vi "Numeric Functions.vi"() -> ()   [LabVIEW 2023]
doc: "This example shows how the Add function operates with different data types. These concepts also apply to the Subtract, Multiply, and Divide, Increment, Decrement, Add Array Elements, Multiply Array Elements, Absolute Value, Round To Nearest, Round To -Infinity, Round To +Infinity, Scale By Power, Square Root, Square, Negate, Reciprocal, and Sign functions."
uses:
  <vilib>/silver_ctls/ArrayMatrixCluster/Real Matrix NI_Silver.ctl
  <vilib>/Analysis/Matrix/Numeric/Add/Add - RM,RM.vi
  <vilib>/Analysis/Matrix/NI_Matrix.lvlib
panel:
  in  "Tab Control":T1(tab)
  in  "Numeric Addend 2":dbl=2.0
  in  "Numeric Addend 1":dbl=1.0
  out "Numeric Sum":dbl
  out "Array Sum":dbl[](array[numeric])
  in  "Array Addend 2":dbl[](array[numeric])=[10.0, 11.0, 12.0, 13.0]
  in  "Array Addend 1":dbl[](array[numeric])=[0.0, 1.0, 2.0]
  out "Array Sum":dbl[](array[numeric])
  in  "Array Addend":dbl[](array[numeric])=[0.0, 1.0, 2.0]
  in  "Numeric Addend":dbl=10.0
  out "Real Matrix Sum":T2
  in  "Real Matrix Addend 2":T2=[[10.0, 11.0, 12.0], [13.0, 14.0, 15.0], [16.0, 17.0, 18.0]]
  in  "Real Matrix Addend 1":T2=[[0.0, 1.0, 2.0], [3.0, 4.0, 5.0], [6.0, 7.0, 8.0]]
  out "Cluster Result":T3
  in  "Cluster Addend 2":T3={"Numeric Addend 1"=1.0, "Numeric Addend 1"=2.0, "Array Addend"=[10.0, 11.0]}
  in  "Cluster Addend 1":T3={"Numeric Addend 1"=1.0, "Numeric Addend 1"=2.0, "Array Addend"=[0.0, 1.0]}
  out "Cluster Result":T3
  in  "Cluster Addend":T3={"Numeric Addend 1"=1.0, "Numeric Addend 1"=2.0, "Array Addend"=[3.0, 4.0]}
  in  "Numeric Addend":i32=10
  in  "Numeric":dbl=60.5
  out "Time Stamp Control":timestamp
  out "Time Stamp Control 2":timestamp
  # "Overview: Demonstrates how the Add function operates with different data types.\nInstructions:\n1. Run the VI.\n2. Examine the different cases.\n3. Although this example demonstrates the Add function, the concepts also apply to other Numeric functions, including the Compound Arithmetic function which can do numeric operations on more than two inputs."
  # "+"
  # "="
  # "The Add function computes a simple numeric sum for two numeric datatypes."
  # "+"
  # "="
  # "Arrays can be added using the add function as well.  The result is an array of sums of each value in the addend arrays. If the arrays have different numbers of elements, the size of their sum will be the smaller of the two arrays."
  # "+"
  # "="
  # "A numeric added to an array results in the addition of the numeric to each item in the array."
  # "+"
  # "="
  # "Matrices can be added using the add function.  Simply wire in your matrices to the function to compute the matrix sum."
  # "+"
  # "="
  # "Adding Cluster datatypes results in the pair-wise addition of each element in the addend clusters.  The clusters must have the same number of elements and the corresponding elements must have compatible datatypes to use the Add function."
  # "+"
  # "="
  # "Adding a numeric to a cluster results in the addition of the numeric to each element in the cluster."
  # "+"
  # "="
  # "Numbers can be added with Timestamps to result in a timestamp representing the timestamp + \"Numeric\" seconds."
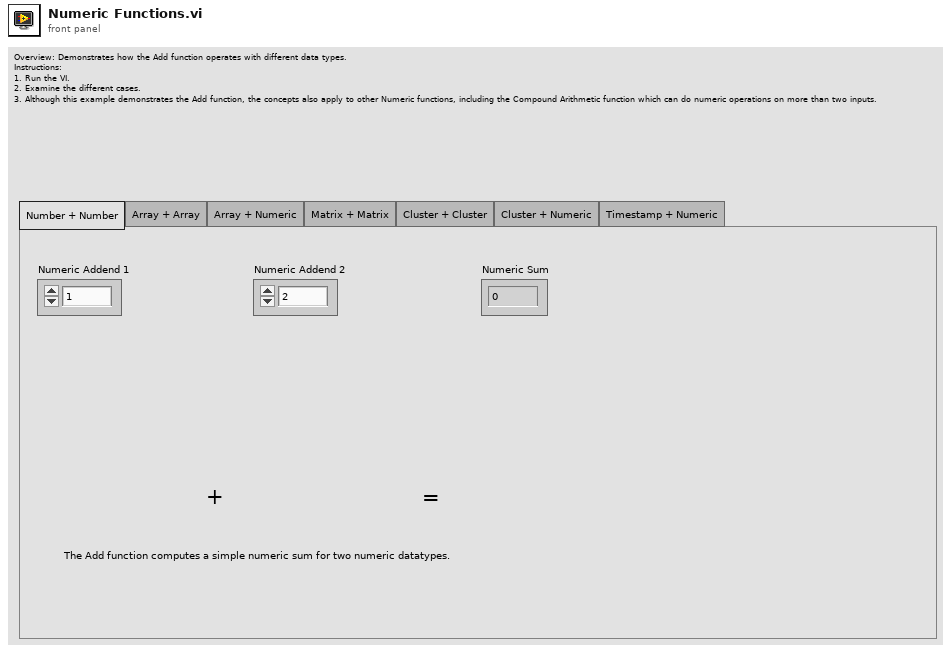
[diagram p1: front panel]
types:
  T1 = enum32{"Number + Number", "Array + Array", "Array + Numeric", "Matrix + Matrix", "Cluster + Cluster", "Cluster + Numeric", "Timestamp + Numeric"}
  T2 = typedef "Real Matrix NI_Silver.ctl" = dbl[][]
  T3 = cluster{"Numeric Addend 1":dbl, "Numeric Addend 1":dbl, "Array Addend":dbl[]}
  T4 = typedef "NI_Matrix.lvlib/RealMatrix.ctl" = dbl[][]
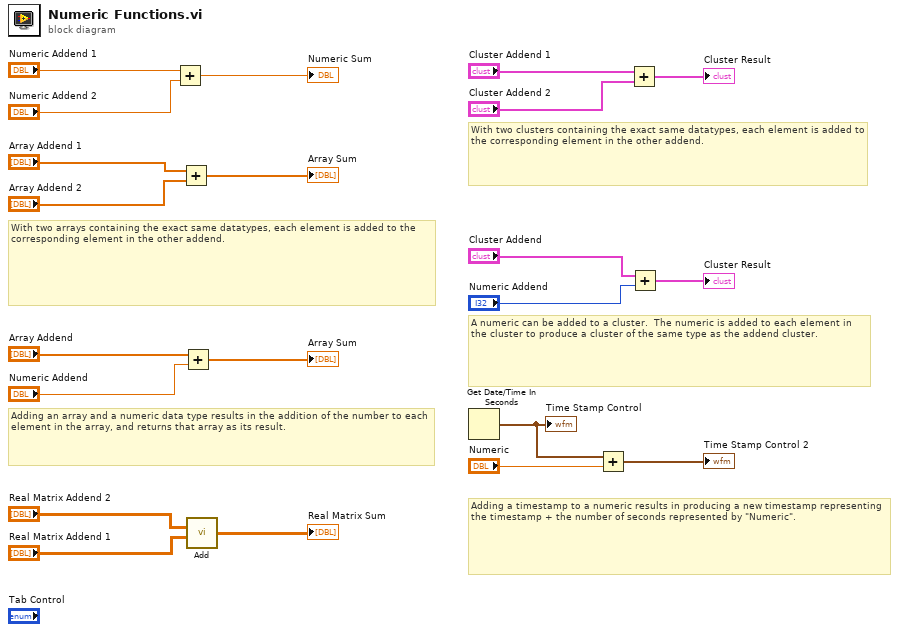
[diagram p0: block diagram]
diagram:
  # "With two arrays containing the exact same datatypes, each element is added to the corresponding element in the other addend."
  # "Adding a timestamp to a numeric results in producing a new timestamp representing the timestamp + the number of seconds represented by \"Numeric\"."
  # "Adding an array and a numeric data type results in the addition of the number to each element in the array, and returns that array as its result."
  # "A numeric can be added to a cluster.  The numeric is added to each element in the cluster to produce a cluster of the same type as the addend cluster."
  # "With two clusters containing the exact same datatypes, each element is added to the corresponding element in the other addend."
  n1 = Add(x="Numeric Addend 1", y="Numeric Addend 2") -> (x+y=→"Numeric Sum":dbl)
  n2 = Add(x="Array Addend 1", y="Array Addend 2") -> (x+y=→"Array Sum":dbl[])
  n3 = Add(x="Array Addend", y="Numeric Addend") -> (x+y=→"Array Sum":dbl[])
  n4 = call-poly <vilib>:"Add.vi"("Real Matrix B"="Real Matrix Addend 1", "Real Matrix A"="Real Matrix Addend 2") -> ("A + B"=→"Real Matrix Sum":T4)
  n5 = Get Date/Time In Seconds() -> (seconds since 1Jan1904=w1:timestamp)
  "Time Stamp Control" <- w1
  n6 = Add(x=w1, y="Numeric") -> (x+y=→"Time Stamp Control 2":timestamp)
  n7 = Add(x="Cluster Addend 1", y="Cluster Addend 2") -> (x+y=→"Cluster Result":T3)
  n8 = Add(x="Cluster Addend", y="Numeric Addend") -> (x+y=→"Cluster Result":T3)
